vi "Get Data Type.vi"(7 "Section":string, 8 "error in (no error)":errorcluster, 10 "Key":string, 11 "config-base in":refnum<class "config-base.lvclass">) -> (0 "error out":errorcluster, 2 "Data Type":T1, 3 "config-base out":refnum<class "config-base.lvclass">)   [LabVIEW 2020, in "hse-config.lvlib" / "config-base.lvclass"]
doc: "Returns the data type of a key.\n\n____\nHAMPEL SOFTWARE ENGINEERING v3.8.0 (2023-12-18 14:41)"
uses:
  config-base.lvclass
  <vilib>/Utility/Data Type/Type Definitions/Data Type.ctl
  config-base.lvclass/config-base.ctl
  <vilib>/Utility/Data Type/NI_Data Type.lvlib
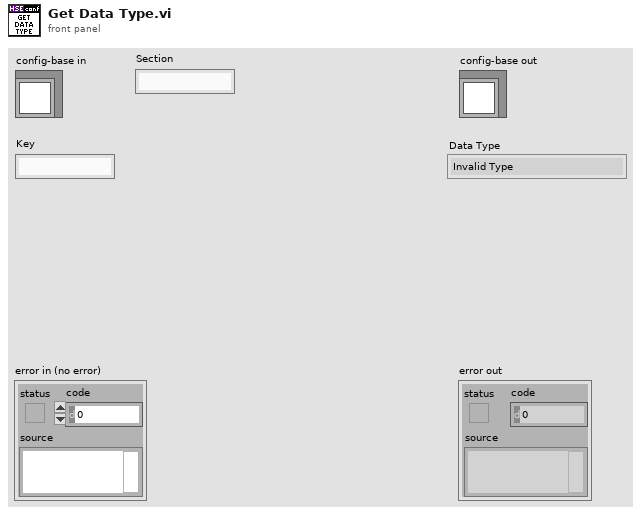
[diagram p1: front panel]
types:
  T1 = typedef "NI_Data Type.lvlib/Data Type.ctl" = enum8{"Invalid Type", "Void", "I8", "I16", "I32", "I64", "U8", "U16", "U32", "U64", "Single Float", "Double Float", "Extended Float", "Single Complex", "Double Complex", "Extended Complex", "Enum U8", "Enum U16", "Enum U32", "Enum U64", "Single Float With Unit", "Double Float With Unit", "Extended Float With Unit", "Single Complex with Unit", "Double Complex with Unit", "Extended Complex with Unit", "Boolean", "String", "Path", "Picture", "Tag", "Array", "Cluster", "Variant", "LV Variant", "Waveform", "Timestamp", "Digital Waveform", "Digital Data", "ExpressData", "Refnum", "External Data", "VI", "Poly VI", "LabVIEW Class Instance", "Fixed Point", "Set Collection", "Map Collection"}
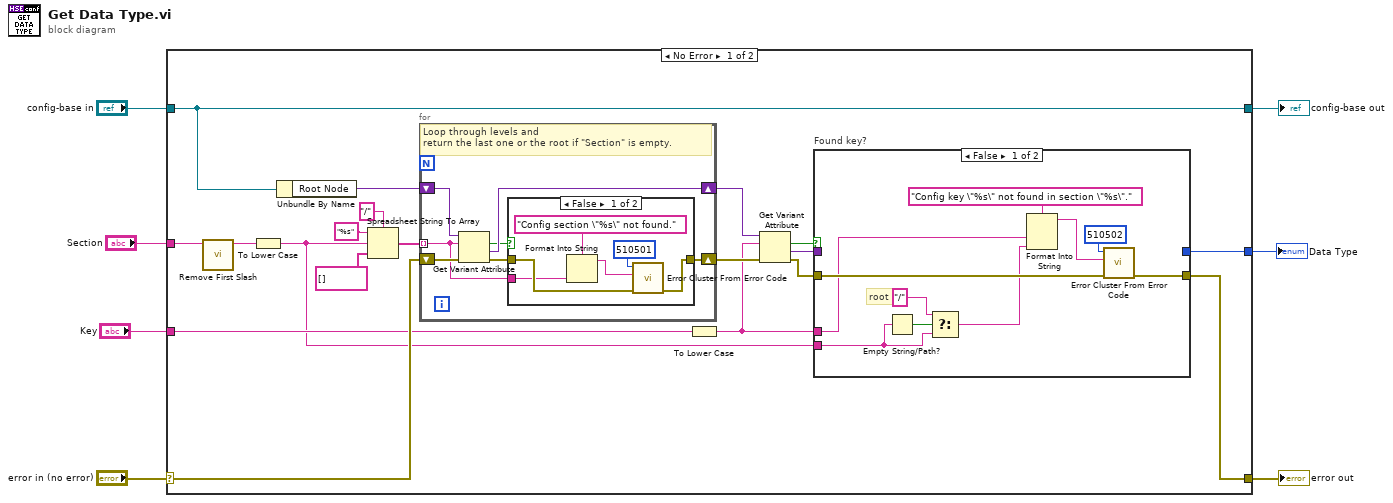
[diagram p0: block diagram]
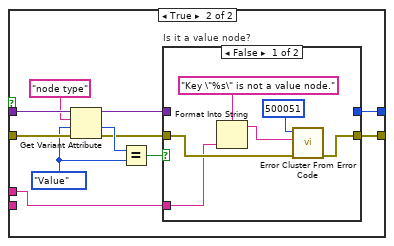
[diagram p2: hidden frame]
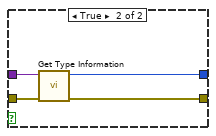
[diagram p3: hidden frame]
diagram:
  n1 = case shown="No Error" "error in (no error)" {
    selector: "error in (no error)" -> [w19 w73]
    tunnel: [w11 w73] -> w6
    tunnel: [w26 w72] -> w4
    tunnel: "config-base in" -> [w26 w72]
    tunnel: "Section" -> [w22 _]
    tunnel: "Key" -> [w13 _]
    tunnel: [w12 _] -> w1
    frame No Error {
      n2 = call "Remove First Slash.vi"("Section"=w22) -> ("result string"=w10:string)  [unwired: 10 in]
      n3 = To Lower Case(string=w10) -> (all lower case string=w8:string)
      n4 = Unbundle By Name(w26) -> ("Root Node"=w20:variant)
      n5 = Spreadsheet String To Array(delimiter (Tab)="/" ("Split Pattern"), format string="%s", spreadsheet string=w8, array type (2D Dbl)=string[] []) -> (array=w21:string[])
      n6 = for {
        shift-right: [w59] -> w17
        shift-left: w19 -> [w63]
        tunnel: w21 -> [w58] mode=indexing
        shift-right: [w62] -> w18
        shift-left: w20 -> [w64]
        # "Loop through levels and\nreturn the last one or the root if \"Section\" is empty."
        n7 = Get Variant Attribute(Variant=w64, name=w58, error in=w63) -> (found=w60:bool, value=w62:variant, error out=w61:errorcluster)  [unwired: 1 in, 1 out]
        n8 = case shown="False" w60 {
          tunnel: w61 -> [w70 w71]
          tunnel: [w69 w71] -> w59
          tunnel: w58 -> [w65 _]
          frame False {
            n9 = Format Into String(format string="Config section \"%s\" not found.", w65) -> (resulting string=w66:string)  [unwired: 2 in, 1 out]
            n10 = call <vilib>:"Error Cluster From Error Code.vi"("error in (no error)"=w70, "error message (\"\")"=w66, "error code (0)"=510501) -> ("error out"=w69:errorcluster)  [unwired: 6 in]
          }
          frame True {
          }
        }
      }
      n11 = To Lower Case(string=w13) -> (all lower case string=w9:string)
      n12 = Get Variant Attribute(Variant=w18, name=w9, error in=w17) -> (found=w16:bool, value=w15:variant, error out=w14:errorcluster)  [unwired: 1 in, 1 out]
      n13 = case "Found key?" shown="False" w16 {
        tunnel: w15 -> [_ w47]
        tunnel: w14 -> [w30 w46]
        tunnel: w9 -> [w28 w39]
        tunnel: [_ w38] -> w12
        tunnel: [w31 w37] -> w11
        tunnel: w8 -> [w27 _]
        frame False {
          # "root"
          n14 = Empty String/Path?(string/path=w27) -> (empty?=w35:bool)
          n15 = Select(t="/", s=w35, f=w27) -> (s? t:f=w29:string)
          n16 = Format Into String(format string="Config key \"%s\" not found in section \"%s\".", w28, w29) -> (resulting string=w34:string)  [unwired: 2 in, 1 out]
          n17 = call <vilib>:"Error Cluster From Error Code.vi"("error in (no error)"=w30, "error message (\"\")"=w34, "error code (0)"=510502) -> ("error out"=w31:errorcluster)  [unwired: 6 in]
        }
        frame True {
          w43 = enum8{"Root", "Section", "Value"}."Value" ("Node Type")
          n18 = Get Variant Attribute(Variant=w47, name="node type", default value (empty Variant)=w43, error in=w46) -> (duplicate Variant=w41:variant, value=w44:enum8{"Root", "Section", "Value"}, error out=w40:errorcluster)  [unwired: 1 out]
          n19 = Equal?(x=w44, y=w43) -> (x = y?=w42:bool)
          n20 = case "Is it a value node?" shown="False" w42 {
            tunnel: w41 -> [_ w57]
            tunnel: w40 -> [w50 w56]
            tunnel: [_ w55] -> w38
            tunnel: w39 -> [w49 _]
            tunnel: [w48 w54] -> w37
            frame False {
              n21 = Format Into String(format string="Key \"%s\" is not a value node.", w49) -> (resulting string=w52:string)  [unwired: 2 in, 1 out]
              n22 = call <vilib>:"Error Cluster From Error Code.vi"("error in (no error)"=w50, "error message (\"\")"=w52, "error code (0)"=500051) -> ("error out"=w48:errorcluster)  [unwired: 6 in]
            }
            frame True {
              n23 = call <vilib>:"Get Type Information.vi"("error in (no error)"=w56, "variant"=w57) -> ("error out"=w54:errorcluster, "type"=w55:T1)  [unwired: 5 in, 3 out]
            }
          }
        }
      }
    }
    frame Error {
    }
  }
  "error out" <- w6
  "config-base out" <- w4
  "Data Type" <- w1
